vi "InRangeCheck&Display_DP_Ver2.1.vi"(1 "Set Pt lower limit":dbl, 4 "Set Pt upper limit":dbl, 5 "Delta range>0":dbl=0.008, 7 "Set Point":dbl, 8 "Sample points (120)":u32=120, 9 "Current value":dbl, 10 "Data Array In":dbl[](array[numeric])) -> (0 "Data Array Out":dbl[](array[numeric]), 2 "Display Cluster":T1 {"STD" format="%.6f"; "RMS" format="%#_4g"}, 3 "Reach to set pt?":bool)   [LabVIEW 2012]
uses:
  <vilib>/Analysis/5stat.llb/RMS (DBL).vi
  <vilib>/Analysis/NI_AALBase.lvlib
  <vilib>/Analysis/NI_AALPro.lvlib
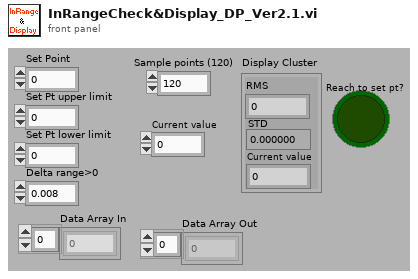
[diagram p1: front panel]
types:
  T1 = cluster{"RMS":dbl, "STD":dbl, "Current value":dbl}
  T2 = cluster{"rms value":dbl, "standard deviation":dbl, "Current value":dbl}
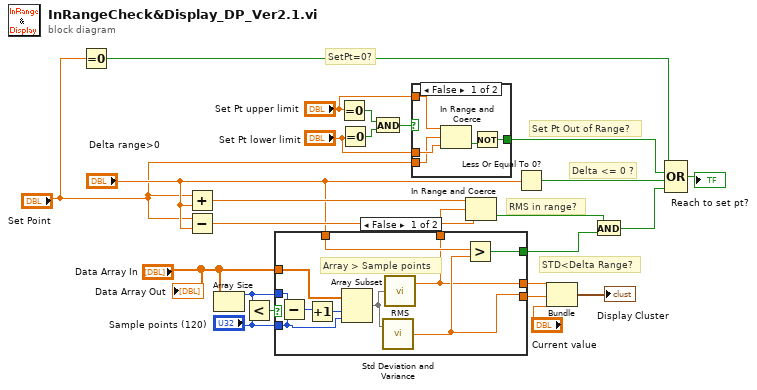
[diagram p0: block diagram]
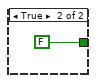
[diagram p2: hidden frame]
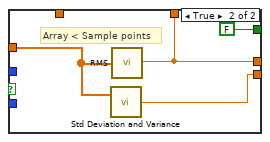
[diagram p3: hidden frame]
diagram:
  # "SetPt=0?"
  # "Delta <= 0 ?"
  # "RMS in range?"
  # "STD<Delta Range?"
  # "Set Pt Out of Range?"
  n1 = Equal To 0?(x="Set Point") -> (x = 0?=w1:bool)
  n2 = Add(x="Set Point", y="Delta range>0") -> (x+y=w25:dbl)
  n3 = Subtract(x="Set Point", y="Delta range>0") -> (x-y=w24:dbl)
  n4 = Array Size(array="Data Array In") -> (size(s)=w16:i32)
  n5 = Less?(x=w16, y="Sample points (120)") -> (x < y?=w18:bool)
  n6 = case shown="False" w18 {
    tunnel: "Sample points (120)" -> [w31 _]
    tunnel: w16 -> [w35 _]
    tunnel: "Data Array In" -> [w30 w38]
    tunnel: [w27 w36] -> w11
    tunnel: [w29 w39] -> w10
    tunnel: "Delta range>0" -> [w28 _]
    tunnel: [w27 w36] -> w13
    tunnel: [w26 FALSE] -> w12
    frame False {
      # "Array > Sample points"
      n7 = Subtract(x=w35, y=w31) -> (x-y=w34:u32)
      n8 = Increment(x=w34) -> (x+1=w32:u32)
      n9 = Array Subset(array=w30, index=w32, length=w31) -> (w33:dbl[])
      n10 = call <vilib>:"Std Deviation and Variance.vi"("X"=w33) -> ("standard deviation"=w29:dbl)  [unwired: 1 in, 2 out]
      n11 = call-poly <vilib>:"RMS.vi"("X"=w33) -> ("rms value"=w27:dbl)  [unwired: 1 out]
      n12 = Greater?(x=w28, y=w29) -> (0:w26:bool)
    }
    frame True {
      # "Array < Sample points"
      n13 = call <vilib>:"Std Deviation and Variance.vi"("X"=w38) -> ("standard deviation"=w39:dbl)  [unwired: 1 in, 2 out]
      n14 = call-poly <vilib>:"RMS.vi"("X"=w38) -> ("rms value"=w36:dbl)  [unwired: 1 out]
    }
  }
  n15 = Equal To 0?(x="Set Pt upper limit") -> (x = 0?=w8:bool)
  n16 = Equal To 0?(x="Set Pt lower limit") -> (x = 0?=w7:bool)
  n17 = And(x=w8, y=w7) -> (x .and. y?=w6:bool)
  n18 = case shown="False" w6 {
    tunnel: "Set Pt upper limit" -> [w43 _]
    tunnel: "Set Pt lower limit" -> [w42 _]
    tunnel: "Set Point" -> [w41 _]
    tunnel: [w40 FALSE] -> w3
    frame False {
      n19 = In Range and Coerce(upper limit=w43, x=w41, lower limit=w42) -> (In Range?=w44:bool)  [unwired: 1 out]
      n20 = Not(x=w44) -> (.not. x?=w40:bool)
    }
    frame True {
    }
  }
  n21 = In Range and Coerce(upper limit=w25, x=w13, lower limit=w24) -> (In Range?=w20:bool)  [unwired: 1 out]
  n22 = Less Or Equal To 0?(x="Delta range>0") -> (x <= 0?=w23:bool)
  n23 = Bundle("rms value"=w11, "standard deviation"=w10, "Current value"="Current value") -> (→"Display Cluster":T2)  [unwired: 1 out]
  n24 = And(x=w20, y=w12) -> (x .and. y?=w19:bool)
  n25 = Compound Arithmetic op=OR(w1, w3, w23, w19) -> (→"Reach to set pt?":bool)
  "Data Array Out" <- "Data Array In"
